vi "Initialize.vi"(8 "error in":errorcluster, 11 "Base Software in":refnum<class "Base Software.lvclass">) -> (0 "error out":errorcluster, 3 "Base Software out":refnum<class "Base Software.lvclass">)   [LabVIEW 2019, in "Base Software.lvlib" / "Main.lvlib" / "Base Software.lvclass"]
uses:
  Project/Base Software.lvclass
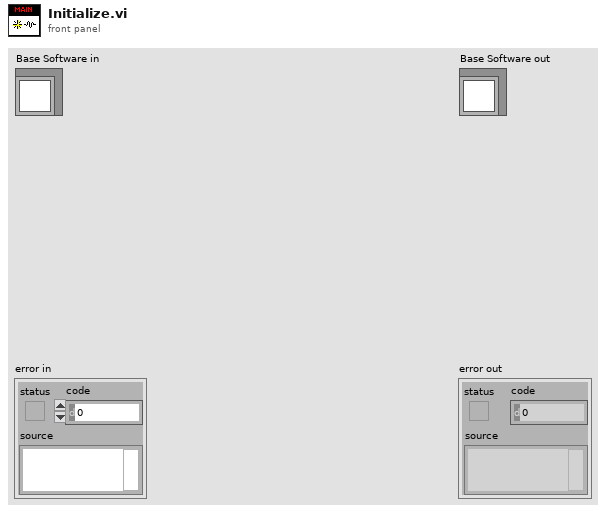
[diagram p1: front panel]
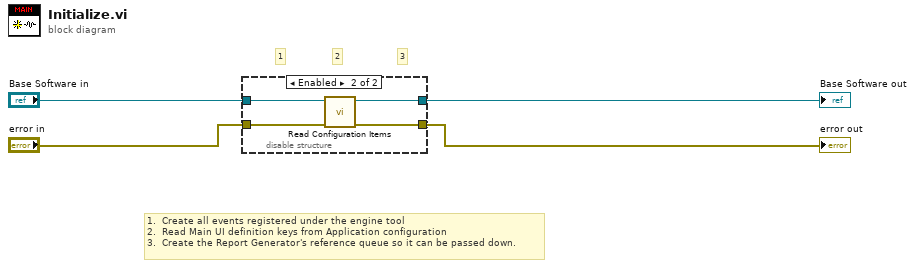
[diagram p0: block diagram]
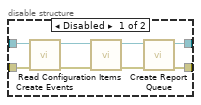
[diagram p2: hidden frame]
diagram:
  # "1.  Create all events registered under the engine tool\n2.  Read Main UI definition keys from Application configuration\n3.  Create the Report Generator's reference queue so it can be passed down."
  # "3"
  # "2"
  # "1"
  n1 = disable-structure shown="Enabled" {
    disable-tunnel: "Base Software in" -> [w12 w16]
    disable-tunnel: "error in" -> [w11 w15]
    disable-tunnel: [w6 w14] -> w2
    disable-tunnel: [w5 w13] -> w1
    frame Disabled {
      n2 = call "Create Events.vi"("error in"=w11, "Base Software in"=w12) -> ("error out"=w9:errorcluster, "Base Software out"=w10:refnum<class "Base Software.lvclass">)  [unwired: 8 in]
      n3 = call "Read Configuration Items.vi"("error in"=w9, "Base Software in"=w10) -> ("error out"=w7:errorcluster, "Base Software out"=w8:refnum<class "Base Software.lvclass">)  [unwired: 8 in]
      n4 = call "Create Report Queue.vi"("error in"=w7, "Base Software in"=w8) -> ("error out"=w5:errorcluster, "Base Software out"=w6:refnum<class "Base Software.lvclass">)  [unwired: 8 in]
    }
    frame Enabled {
      n5 = call "Read Configuration Items.vi"("error in"=w15, "Base Software in"=w16) -> ("error out"=w13:errorcluster, "Base Software out"=w14:refnum<class "Base Software.lvclass">)  [unwired: 8 in]
    }
  }
  "error out" <- w1
  "Base Software out" <- w2
